vi "wrapper.vi"(1 "Parameter":variant[](array[variant])) -> (0 "Result":variant[](array[variant]))   [LabVIEW 2010]
panel:
  out "data":u32
  out "SetupID":u32
  out "waveformType":string
  out "samplingTime":dbl
  out "samplingRate":u32
  out "offset":dbl
  out "amplitude":dbl
  out "frequency":dbl
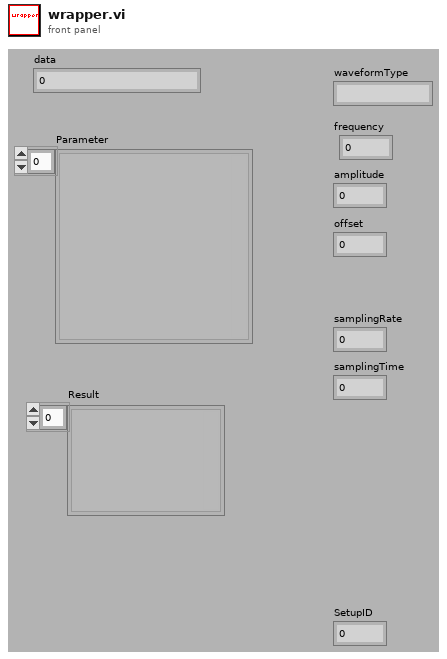
[diagram p1: front panel]
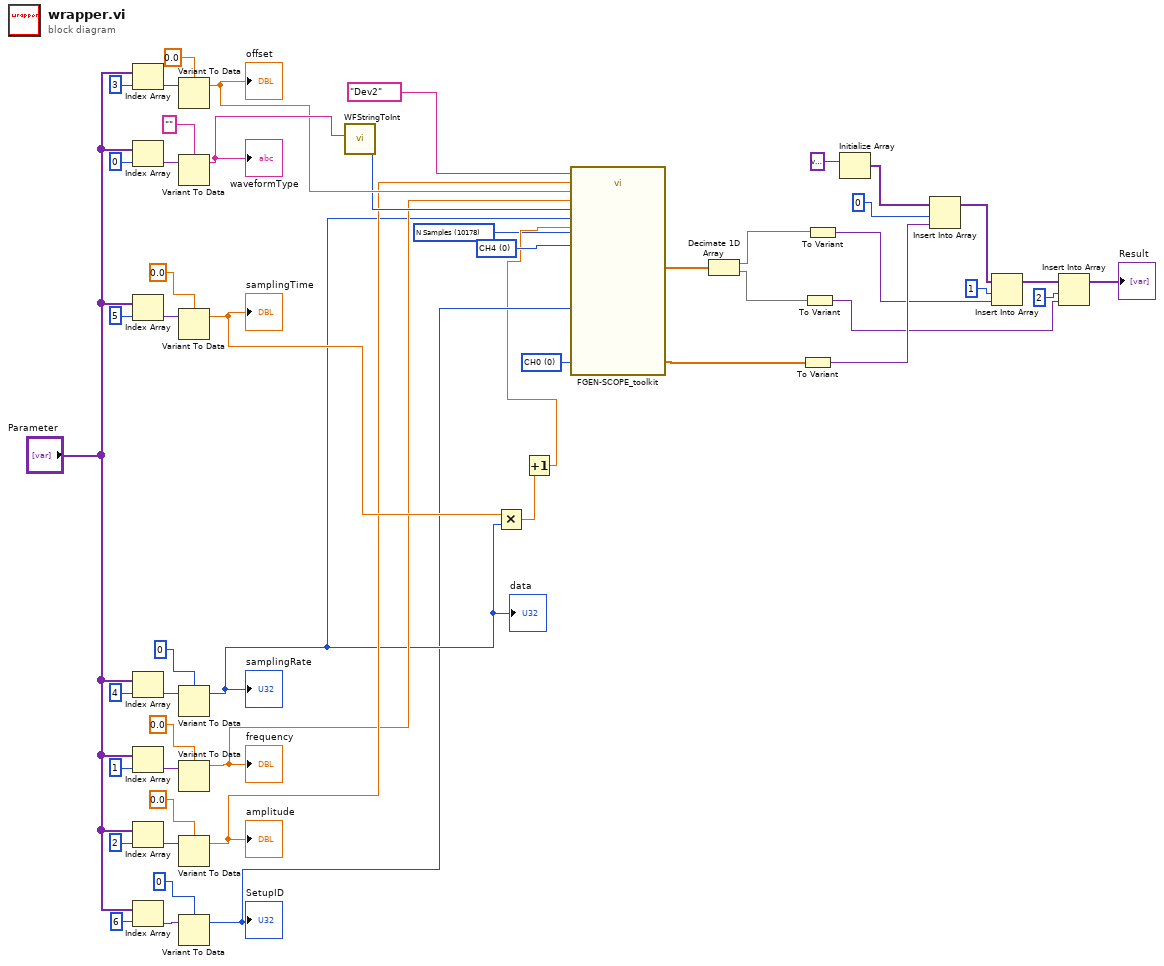
[diagram p0: block diagram]
diagram:
  w1 = u16 10178 items=["N Samples"=10178, "Continuously"=10123] ("Acquire")
  w4 = u16 0 items=["CH4", "CH5", "CH6", "CH7"] ("ChB_Source")
  w5 = u16 0 items=["CH0", "CH1", "CH2", "CH3"] ("ChA_Source")
  n1 = Index Array(array="Parameter", index=3) -> (element=w44:variant)
  n2 = Index Array(array="Parameter", index=0) -> (element=w41:variant)
  n3 = Index Array(array="Parameter", index=5) -> (element=w36:variant)
  n4 = Index Array(array="Parameter", index=4) -> (element=w39:variant)
  n5 = Index Array(array="Parameter", index=1) -> (element=w50:variant)
  n6 = Index Array(array="Parameter", index=2) -> (element=w47:variant)
  n7 = Index Array(array="Parameter", index=6) -> (element=w32:variant)
  n8 = Variant To Data(Variant=w44, type=0.0 ("double precision float")) -> (data=w12:dbl)  [unwired: 1 in, 1 out]
  "offset" <- w12
  n9 = Variant To Data(Variant=w41, type="") -> (data=w33:string)  [unwired: 1 in, 1 out]
  "waveformType" <- w33
  n10 = Variant To Data(Variant=w36, type=0.0 ("double precision float")) -> (data=w14:dbl)  [unwired: 1 in, 1 out]
  "samplingTime" <- w14
  n11 = Variant To Data(Variant=w39, type=u32 0 ("double precision float")) -> (data=w8:u32)  [unwired: 1 in, 1 out]
  "samplingRate" <- w8
  "data" <- w8
  n12 = Variant To Data(Variant=w50, type=0.0 ("double precision float")) -> (data=w9:dbl)  [unwired: 1 in, 1 out]
  "frequency" <- w9
  n13 = Variant To Data(Variant=w47, type=0.0 ("double precision float")) -> (data=w10:dbl)  [unwired: 1 in, 1 out]
  "amplitude" <- w10
  n14 = Variant To Data(Variant=w32, type=u32 0 ("double precision float")) -> (data=w7:u32)  [unwired: 1 in, 1 out]
  "SetupID" <- w7
  n15 = call "WFStringToInt.vi"("WaveFormType"=w33) -> ("WaveFormTypeInt"=w11:u16)  [unwired: 10 in]
  n16 = Multiply(x=w14, y=w8) -> (x*y=w3:dbl)
  n17 = Increment(x=w3) -> (x+1=w2:dbl)
  n18 = call "FGEN-SCOPE_toolkit.vi"("Device Name"=tag "Dev2", "Amplitude"=w10, "DC Offset"=w12, "Frequency"=w9, "Waveform Type"=w11, "Sample Rate (Hz)"=w8, "Record Length"=w2, "Acquire"=w1, "ChA_Source"=w5, "ChB_Source"=w4, "SetupID"=w7) -> ("interleaved array"=w20:dbl[], "time vector"=w21:dbl[])  [unwired: 14 in, 1 out]
  n19 = Decimate 1D Array(w20) -> (w19:dbl[], w18:dbl[])
  n20 = To Variant(anything=w21) -> (Variant=w17:variant)
  n21 = To Variant(anything=w18) -> (Variant=w15:variant)
  n22 = To Variant(anything=w19) -> (Variant=w16:variant)
  n23 = Initialize Array(variant ("variant")) -> (w27:variant[])  [unwired: 1 in]
  n24 = Insert Into Array(array=w27, index=0, new element=w17) -> (w26:variant[])
  n25 = Insert Into Array(array=w26, index=1, new element=w16) -> (w24:variant[])
  n26 = Insert Into Array(array=w24, index=2, new element=w15) -> (→"Result":variant[])
